vi "reshape data.vi"(7 "Status":T2 {"Setting"."X Pos." scale=-2.0..2.0; "Setting"."Y Pos." scale=-2.0..2.0}, 9 "line #":i32, 10 "Effective lines":dbl[][](array[numeric]), 11 "Image输入":T1) -> (3 "Image输出":T1)   [LabVIEW 2013]
uses:
  init & communication/init-status.ctl
  init & communication/Setting.ctl
  init & communication/event-package.ctl
  init & communication/Event1.ctl
  init & communication/data-package.ctl
  init & communication/Event.ctl
  Image.ctl
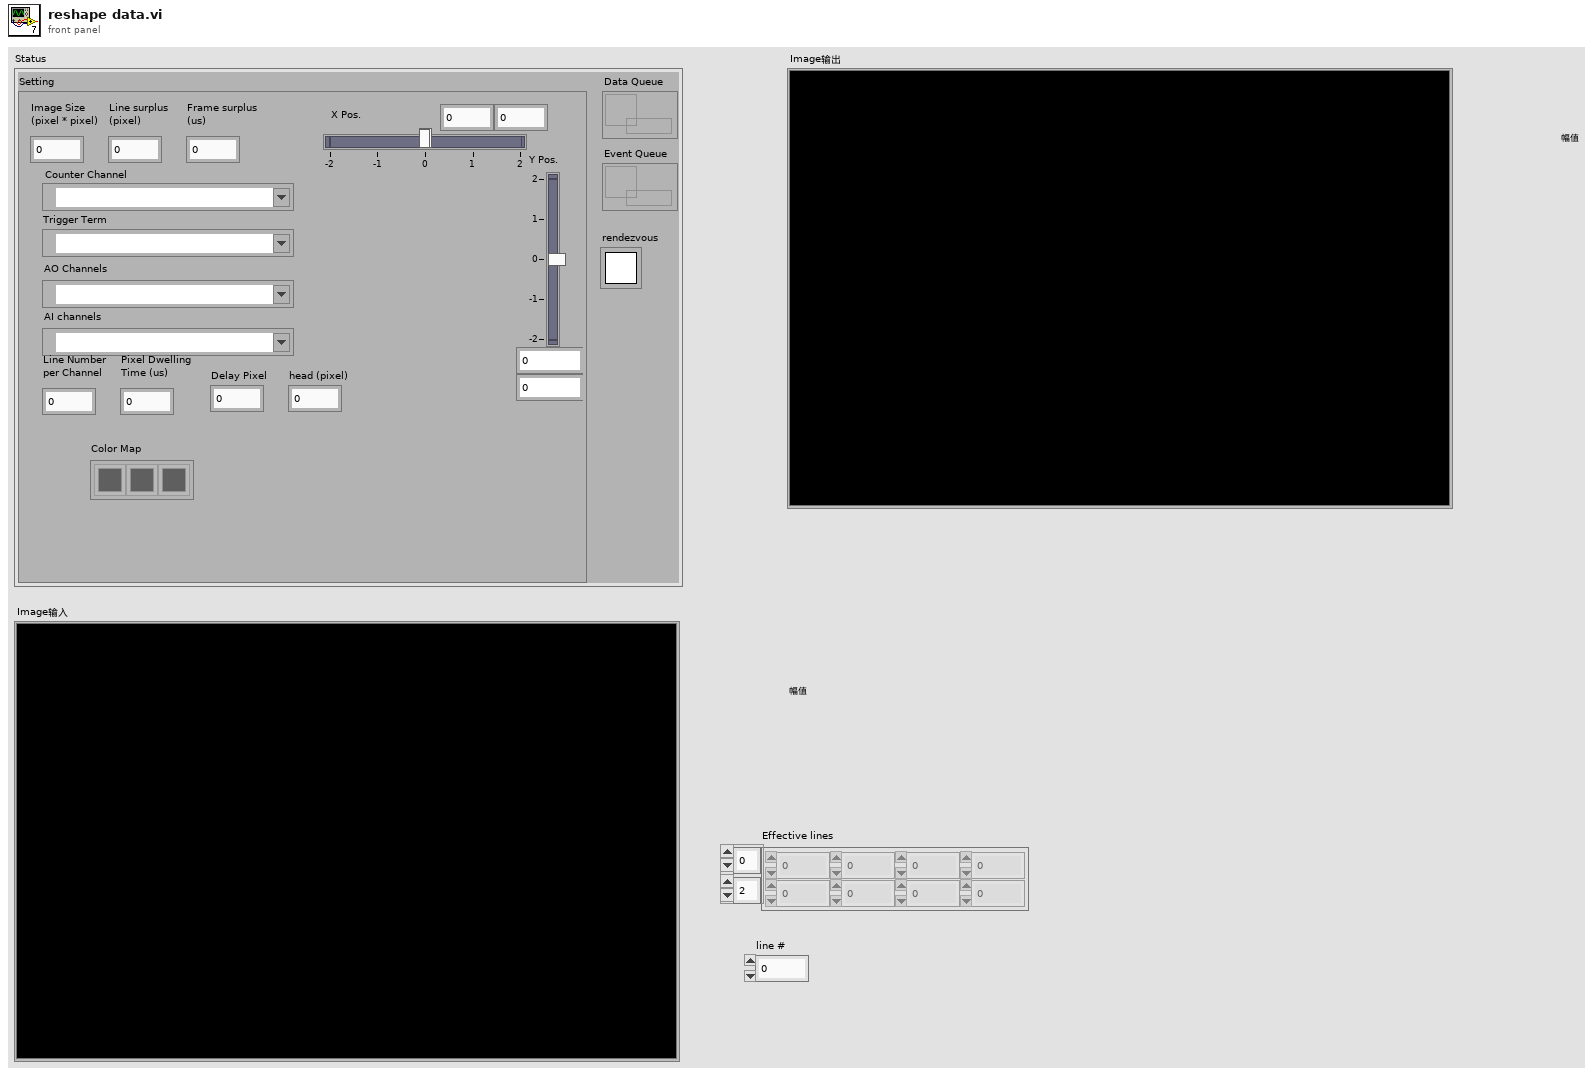
[diagram p1: front panel]
types:
  T1 = typedef "Image.ctl" = dbl[][]
  T2 = typedef "init-status.ctl" = cluster{"Setting":T3, "Event Queue":refnum<queue>, "Data Queue":refnum<queue>, "rendezvous":T4}
  T3 = typedef "Setting.ctl" = cluster{"Image Size\n(pixel * pixel)":i32, "Counter Channel":tag, "Trigger Term":tag, "AO Channels":tag, "Y Pos.":cluster{dbl, dbl}, "X Pos.":cluster{dbl, dbl}, "Line surplus\n(pixel)":i32, "Frame surplus\n(us)":i32, "AI channels":tag, "Line Number\nper Channel":i32, "Delay Pixel":i32, "Pixel Dwelling\nTime (us)":i32, "Color Map":u32[], "head (pixel)":i32}
  T4 = typedef "Rendezvous RefNum" = refnum<k1>
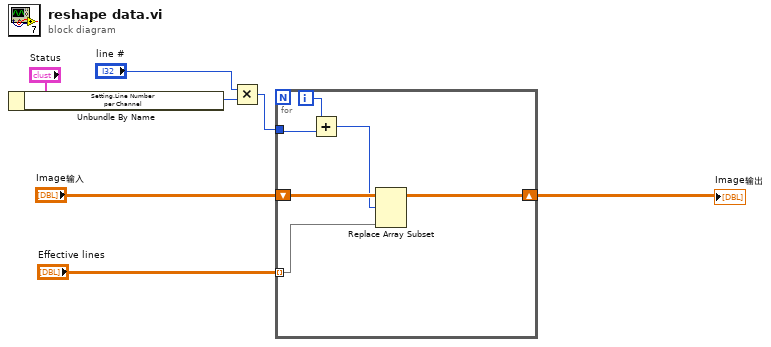
[diagram p0: block diagram]
diagram:
  n1 = Unbundle By Name("Status") -> ("Setting.Line Number\nper Channel"=w4:i32)
  n2 = Multiply(x="line #", y=w4) -> (x*y=w2:i32)
  n3 = for {
    shift-right: [w12] -> w6
    shift-left: "Image输入" -> [w13]
    tunnel: "Effective lines" -> [w8] mode=indexing
    tunnel: w2 -> [w10]
    i -> [w11]
    n4 = Add(x=w11, y=w10) -> (x+y=w9:i32)
    n5 = Replace Array Subset(array=w13, new element=w8, index (row)=w9) -> (w12:T1)  [unwired: 1 in]
  }
  "Image输出" <- w6
